vi "Breaker Enable Logic.vi"(7 "Breaker Enable In":bool, 9 "Reset":bool, 10 "Fault OK":bool, 11 "Breaker Error":u64) -> (1 "Resetting":bool, 2 "Breaker First Error":u64, 3 "Breaker Enable Out":bool)   [LabVIEW 2018]
doc: "Author: Scott Hannahs <sth@magnet.fsu.edu>\nCopyright 2018 Florida State University, All rights reserved."
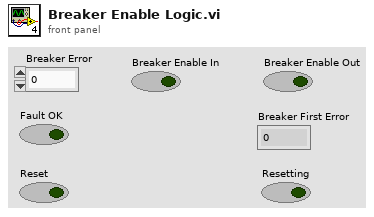
[diagram p1: front panel]
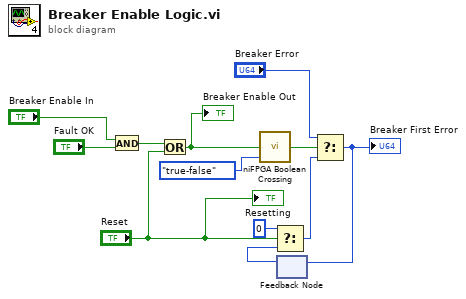
[diagram p0: block diagram]
diagram:
  n1 = And(x="Breaker Enable In", y="Fault OK") -> (x .and. y?=w4:bool)
  n2 = Or(x=w4, y="Reset") -> (x .or. y?=w2:bool)
  "Breaker Enable Out" <- w2
  n3 = call <vilib>:"niFPGA Boolean Crossing.vi"("input"=w2, "direction"=enum8{"either", "false-true", "true-false"}."true-false") -> ("crossing"=w7:bool)  [unwired: 7 in]
  n4 = feedback #1() -> (w10:u64)  [unwired: 1 in]
  n5 = Select(t=u64 0, s="Reset", f=w10) -> (s? t:f=w11:u64)
  n6 = Select(t="Breaker Error", s=w7, f=w11) -> (s? t:f=w9:u64)
  "Breaker First Error" <- w9
  n7 = feedback-in #1(w9) -> ()
  "Resetting" <- "Reset"
